vi "demo.run.HostToFpgaTests.vi"(8 "error in":errorcluster, 11 "filter(s)":string[](array[string])=["hostToFpgaTests"]) -> (0 "error out":errorcluster)   [LabVIEW 2022 SP3]
panel:
  out "Results.out":T1
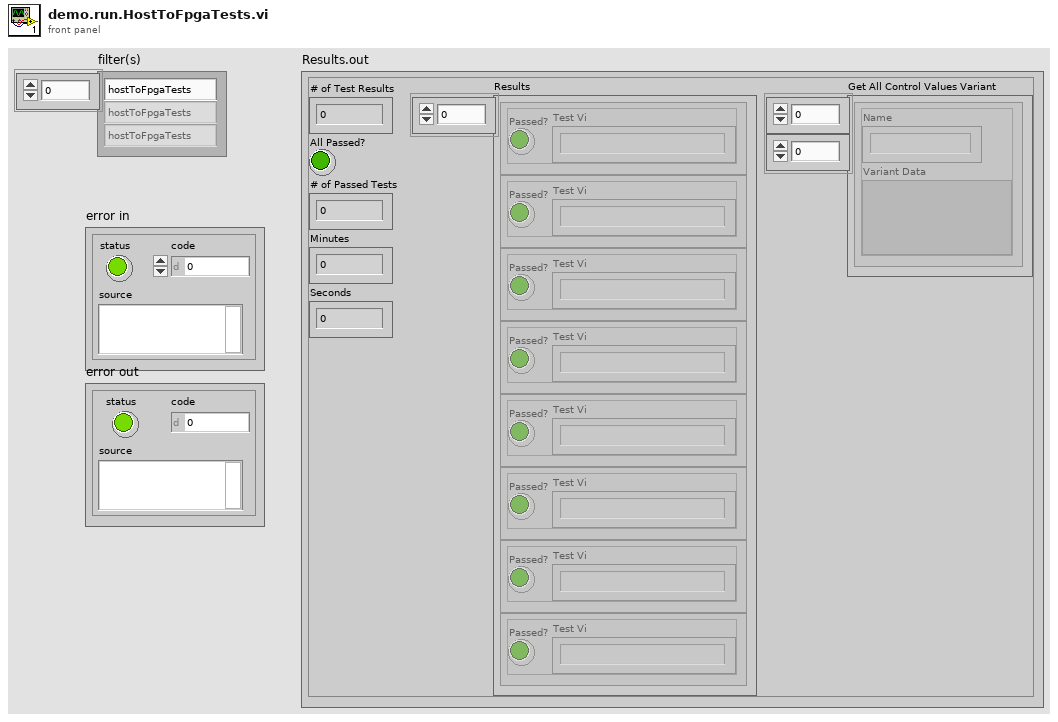
[diagram p1: front panel]
types:
  T1 = cluster{"Results":cluster{"Test Vi":string, "Passed?":bool}[], "# of Test Results":i32, "All Passed?":bool, "# of Passed Tests":i32, "Minutes":u32, "Seconds":u32, "Get All Control Values Variant":cluster{"Name":string, "Variant Data":variant}[][]}
  T2 = cluster{"filter(s)":string[], "path":path, "error in":errorcluster}
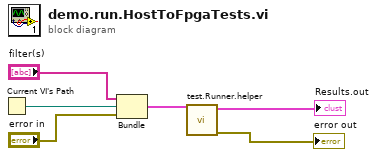
[diagram p0: block diagram]
diagram:
  n1 = Current VI's Path() -> (path=w3:path)
  n2 = Bundle("filter(s)"="filter(s)", "path"=w3, "error in"="error in") -> (w4:T2)  [unwired: 1 in]
  n3 = call "test.Runner.helper.vi"("Parameters.in"=w4) -> ("error out"=→"error out":errorcluster, "Results.out"=→"Results.out":T1)  [unwired: 9 in]
